vi "main.vi"() -> ()   [LabVIEW 2016]
panel:
  out "Title":string="Inventory Check"
  in  "Open report file?":bool=TRUE
  in  "Stop Button":bool
  in  "Run":bool
  in  "Report file path:":path=path "C:/Users/emanu/Desktop/report.xlsx"
  in  "QuickBook file:":path=path "C:/Users/emanu/Desktop/COSMED Asia-Pacific Pty Ltd_ProductServiceList.xlsx"
  in  "Storage file:":path=path "X:/UtilityFiles/Storage.xlsx"
  out "bar":string="You need to double check some items in the inventory in the file: C:\\Users\\emanu\\Desktop\\report.xlsx\r\n\r\nTraceback (most recent call last):\r\n  File \"InventoryCheck.py\", line 43, in <module>\r\n    fileManager.columnAdjustment(reportPath)\r\n  File \"D:\\InventoryCheck\\fileController\\fileManager.py\", line 121, in columnAdjustment\r\n    ws.cell(row = i).style.border.bottom\r\n  File \"C:\\Python34\\lib\\site-packages\\openpyxl-2.5.0a2-py3.4.egg\\openpyxl\\worksheet\\worksheet.py\", line 301, in cell\r\n    raise InsufficientCoordinatesException(msg)\r\nopenpyxl.utils.exceptions.InsufficientCoordinatesException: You have to provide a value either for 'coordinate' or for 'row' *and* 'column'\r\n\r\n"
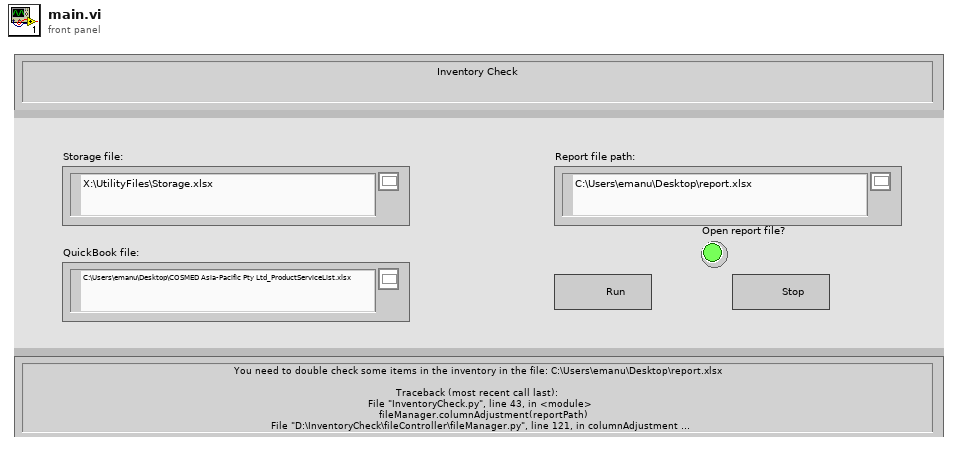
[diagram p1: front panel]
types:
  T1 = cluster{"Excel._Application":refnum<k7>, "Workbooks":refnum<k7>}
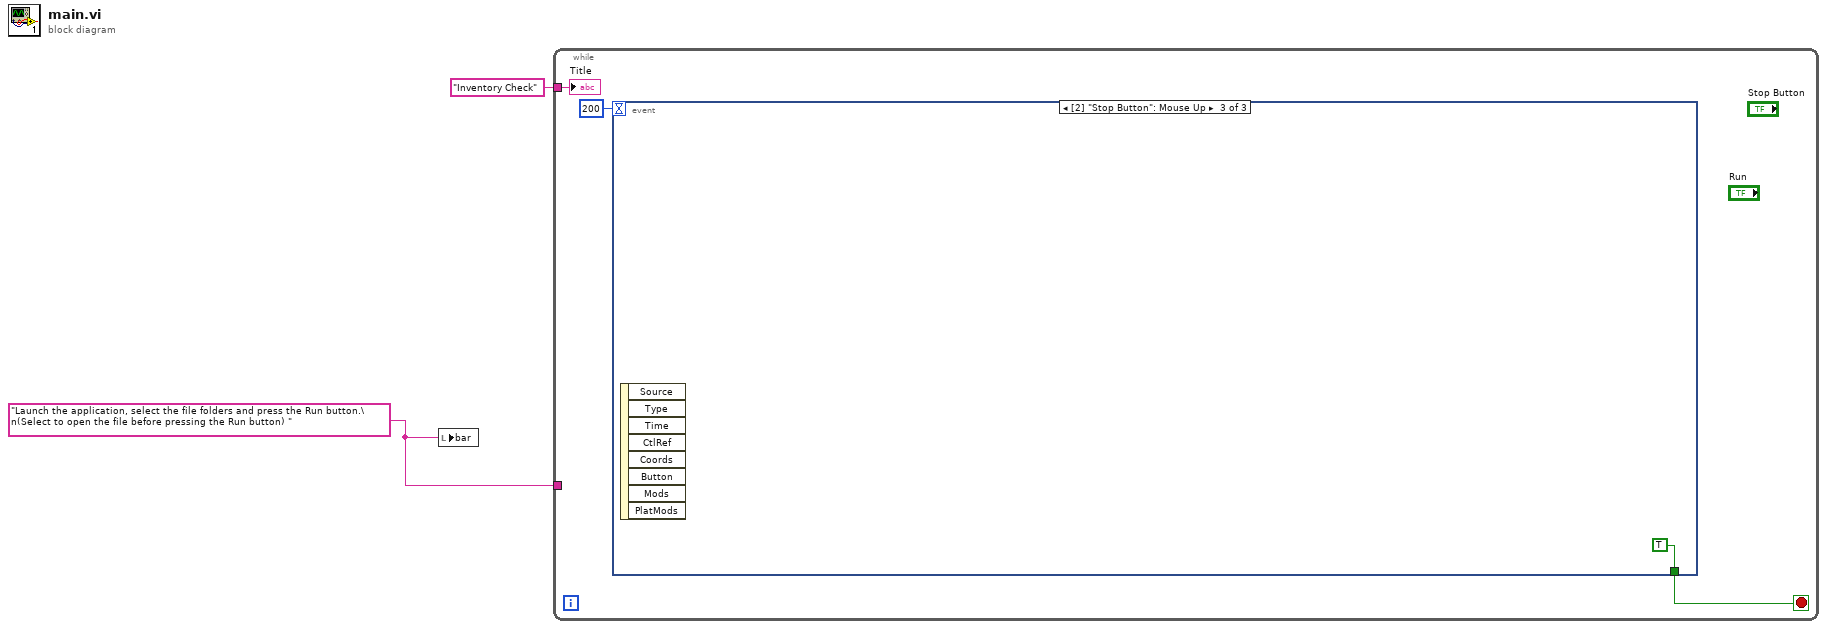
[diagram p0: block diagram]
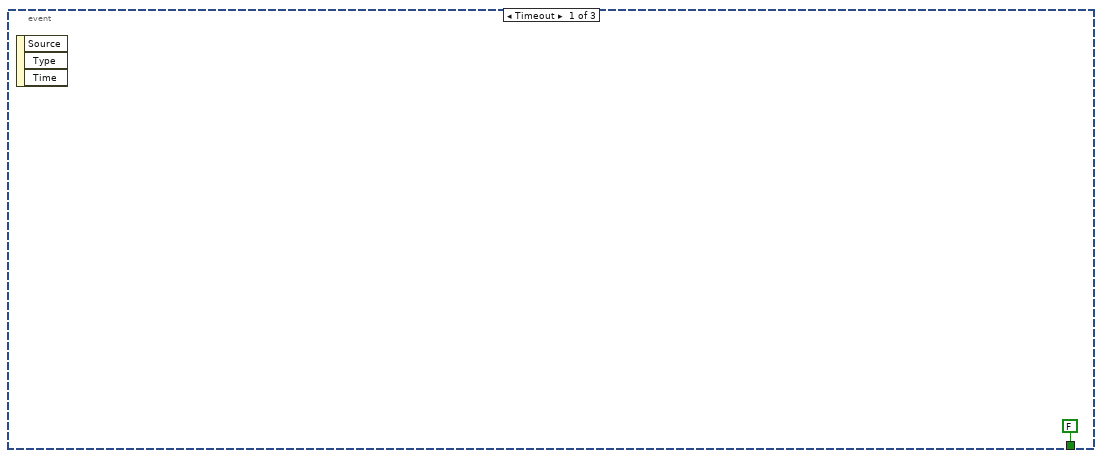
[diagram p2: hidden frame]
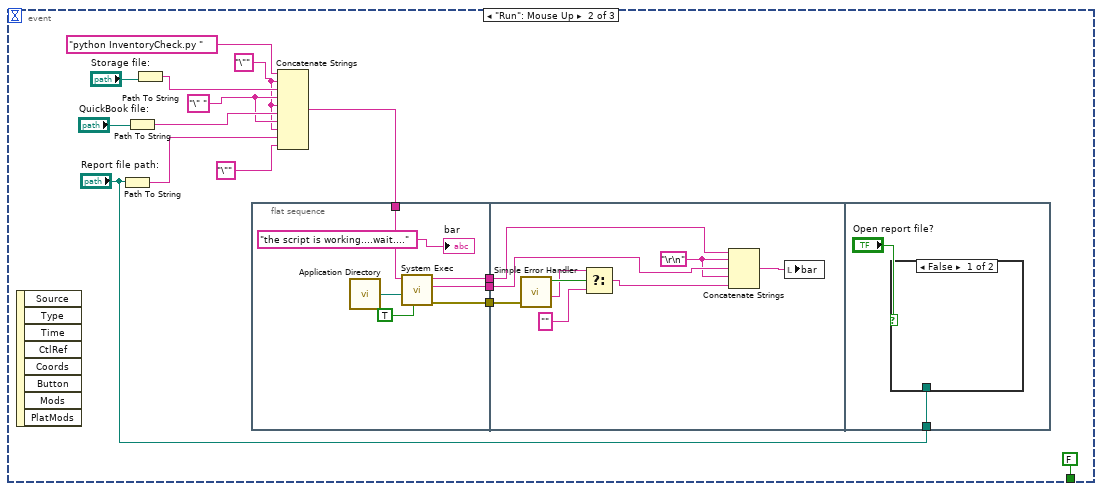
[diagram p3: hidden frame]
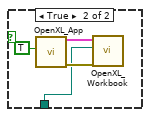
[diagram p4: hidden frame]
diagram:
  w1 = "Launch the application, select the file folders and press the Run button.\n(Select to open the file before pressing the Run button) " ("Title")
  n1 = local write "bar"(w1) -> ()
  n2 = while {
    tunnel: "Inventory Check" ("Title") -> [w3]
    tunnel: w1 -> [_]
    stop <- w5 stop-if-true
    n3 = event shown="[2] \"Stop Button\": Mouse Up" {
      selector: _ -> [_ _ _]
      dyn-events: _ -> [_ _ _]
      timeout: 200 -> [_ _ _]
      tunnel: [FALSE FALSE TRUE] -> w5
      event Timeout {
        n4 = event-data() -> ()  [unwired: 1 in, 3 out]
      }
      event "Run": Mouse Up {
        w14 = "\" " ("string")
        w13 = "\"" ("string")
        n5 = event-data() -> ()  [unwired: 1 in, 8 out]
        n6 = Path To String(path="Report file path:") -> (string=w12:string)
        n7 = Path To String(path="QuickBook file:") -> (string=w15:string)
        n8 = Path To String(path="Storage file:") -> (string=w17:string)
        n9 = flat-sequence {
          tunnel: w20 -> [w28]
          tunnel: [w24] -> w10
          tunnel: [w23] -> w9
          tunnel: [w22] -> w8
          tunnel: w10 -> [w37]
          tunnel: w9 -> [w33]
          tunnel: w8 -> [w32]
          tunnel: "Report file path:" -> [w38]
          frame #0 {
            n10 = call <vilib>:"Application Directory.vi"() -> ("Application Directory"=w27:path)
            n11 = call <vilib>:"System Exec.vi"("run minimized? (F)"=TRUE, "working directory"=w27, "command line"=w28) -> ("error out"=w24:errorcluster, "standard error"=w22:string, "standard output"=w23:string)  [unwired: 3 in, 3 out]
            "bar" <- "the script is working....wait...." ("bar")
          }
          frame #1 {
            w31 = "\r\n"
            n12 = call <vilib>:"Simple Error Handler.vi"("error in (no error)"=w37) -> ("error?"=w36:bool, "source out"=w35:string)  [unwired: 1 in, 6 out]
            n13 = Select(t=w35, s=w36, f="") -> (s? t:f=w30:string)
            n14 = Concatenate Strings(w33, w31, w32, w31, w30) -> (w29:string)
            n15 = local write "bar"(w29) -> ()
          }
          frame #2 {
            n16 = case shown="False" "Open report file?" {
              tunnel: w38 -> [_ w42]
              frame False {
              }
              frame True {
                n17 = call <userlib>:"OpenXL_App.vi"("Visible"=TRUE) -> ("error out"=w43:errorcluster, "Refnum Cluster"=w41:T1)  [unwired: 9 in]
                n18 = call <userlib>:"OpenXL_Workbook.vi"("error in"=w43, "path"=w42, "Refnum Cluster In"=w41) -> ()  [unwired: 7 in, 2 out]
              }
            }
          }
        }
        n19 = Concatenate Strings("python InventoryCheck.py " ("command line"), w13, w17, w14, w13, w15, w14, w13, w12, "\"" ("string")) -> (w20:string)
      }
      event "Stop Button": Mouse Up {
        n20 = event-data() -> ()  [unwired: 1 in, 8 out]
      }
    }
    "Title" <- w3
  }
